vi "DFD Get Zero-Pole-Gain.vi"(7 "type (FLP)":enum16{"FLP", "FXP"}(ring), 8 "error in (no error)":errorcluster, 11 "filter in":T1={"mSRate_Fs"=1.0, "mSRate_Version"="2.0", "mSRate_Comments"="", "mSRate_OrgCoef"={"type"=enum."Undefined", "gain"=1.0, "coef a (k)"=[], "coef b (v)"=[]}, "mSRate_CurCoef"={"type"=enum."Undefined", "gain"=1.0, "coef a (k)"=[], "coef b (v)"=[]}, "mSRate_Quantized?"=FALSE, "mSRate_QCoef"={"type"=enum."Undefined", "gain"=1.0, "coef a (k)"=[], "coef b (v)"=[]}, "mSRate_QSettings"=[], "mSRate_Order"=0, "mSRate_Scaling"={"mSRate_ScaleByPowerOf2?"=FALSE, "mSRate_ScaleType"=enum."No Norm"}} {"mSRate_QSettings"."source" items=["Coef a/k"=0, "Coef b/v"=7, "Input"=1, "Output"=2, "Multiplicand"=3, "Product"=4, "Sum"=5, "Delay"=6, "Gain"=8]}) -> (0 "error out":errorcluster, 1 "poles":cdb[](array[numeric]) format="%.2f", 2 "zeroes":cdb[](array[numeric]) format="%.2f", 3 "filter out":T1={"mSRate_Fs"=1.0, "mSRate_Version"="2.0", "mSRate_Comments"="", "mSRate_OrgCoef"={"type"=enum."Undefined", "gain"=1.0, "coef a (k)"=[], "coef b (v)"=[]}, "mSRate_CurCoef"={"type"=enum."Undefined", "gain"=1.0, "coef a (k)"=[], "coef b (v)"=[]}, "mSRate_Quantized?"=FALSE, "mSRate_QCoef"={"type"=enum."Undefined", "gain"=1.0, "coef a (k)"=[], "coef b (v)"=[]}, "mSRate_QSettings"=[], "mSRate_Order"=0, "mSRate_Scaling"={"mSRate_ScaleByPowerOf2?"=FALSE, "mSRate_ScaleType"=enum."No Norm"}} {"mSRate_QSettings"."source" items=["Coef a/k"=0, "Coef b/v"=7, "Input"=1, "Output"=2, "Multiplicand"=3, "Product"=4, "Sum"=5, "Delay"=6, "Gain"=8]}, 5 "gain":dbl format="%.2f")   [LabVIEW 2017, in "NI_DigFilterLicensed.lvlib"]
doc: "Retrieves the zeroes, poles, and gain (ZPK) of a filter."
uses:
  <vilib>/addons/Digital Filter Design/NI_DigFilterLicensed.lvlib
  <vilib>/addons/Digital Filter Design/_Objects.llb/DFD Filter Obj.ctl
  <vilib>/addons/Digital Filter Design/_Objects.llb/DFD Filter Coef.ctl
  <vilib>/addons/Digital Filter Design/_Objects.llb/DFD Filter Structure Type Selector.ctl
  <vilib>/addons/Digital Filter Design/_Objects.llb/dfd_Internal Quantization Settings.ctl
  <vilib>/addons/Digital Filter Design/_Objects.llb/dfd_Internal Quantization Srcs.ctl
  <vilib>/addons/Digital Filter Design/_Objects.llb/DFD Coef Norm Type.ctl
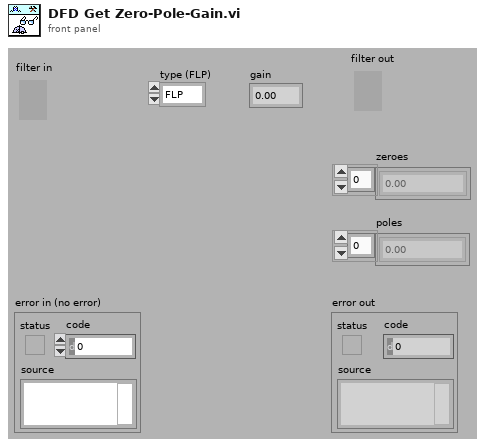
[diagram p1: front panel]
types:
  T1 = typedef "NI_DigFilterLicensed.lvlib/DFD Filter Obj.ctl" = cluster{"mSRate_Fs":dbl, "mSRate_Version":string, "mSRate_Comments":string, "mSRate_OrgCoef":T2, "mSRate_CurCoef":T2, "mSRate_Quantized?":bool, "mSRate_QCoef":T2, "mSRate_QSettings":T4[], "mSRate_Order":i32, "mSRate_Scaling":cluster{"mSRate_ScaleByPowerOf2?":bool, "mSRate_ScaleType":T6}}
  T2 = typedef "NI_DigFilterLicensed.lvlib/DFD Filter Coef.ctl" = cluster{"type":T3, "gain":dbl, "coef a (k)":dbl[], "coef b (v)":dbl[]}
  T3 = typedef "NI_DigFilterLicensed.lvlib/DFD Filter Structure Type Selector.ctl" = enum16{"Undefined", "FIR Direct Form", "FIR Direct Form Transposed", "FIR Symmetric", "FIR Antisymmetric", "IIR Direct Form I", "IIR Direct Form I Transposed", "IIR Direct Form II", "IIR Direct Form II Transposed", "IIR Cascaded Second Order Sections Form I", "IIR Cascaded Second Order Sections Form I Transposed", "IIR Cascaded Second Order Sections Form II", "IIR Cascaded Second Order Sections Form II Transposed", "Lattice Allpass (basic sections)", "Lattice Allpass (one multiplier sections)", "Lattice Allpass (normalized sections)", "Lattice AR (basic sections)", "Lattice AR (one multiplier sections)", "Lattice AR (normalized sections)", "Lattice MA (minimum phase)", "Lattice MA (maximum phase)", "Lattice ARMA (basic sections)", "Lattice ARMA (one multiplier sections)", "Lattice ARMA (normalized sections)"}
  T4 = typedef "NI_DigFilterLicensed.lvlib/dfd_Internal Quantization Settings.ctl" = cluster{"source":T5, "wl":i16, "iwl":i16, "overflow mode":enum16{"Saturation", "Wrap"}, "rounding mode":enum16{"Nearest", "Truncation"}, "signed?":bool}
  T5 = typedef "NI_DigFilterLicensed.lvlib/dfd_Internal Quantization Srcs.ctl" = u16
  T6 = typedef "NI_DigFilterLicensed.lvlib/DFD Coef Norm Type.ctl" = enum16{"No Norm", "Time Domain 1-Norm", "Time Domain 2-Norm", "Time Domain Inf-Norm"}
  T7 = typedef "NI_DigFilterLicensed.lvlib/DFD Filter Structure Id.ctl" = enum16{"Undefined", "FIR", "IIR Direct", "IIR SOS", "IIR Allpass", "IIR AR", "IIR ARMA"}
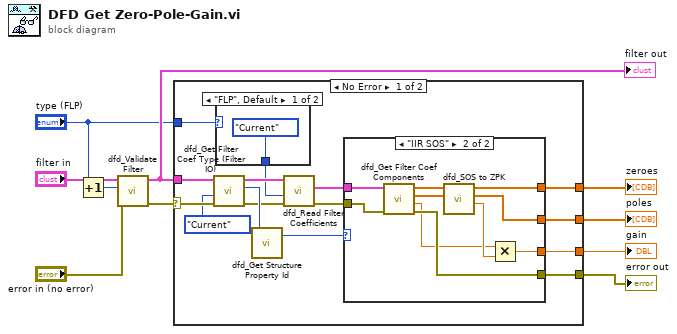
[diagram p0: block diagram]
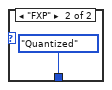
[diagram p2: hidden frame]
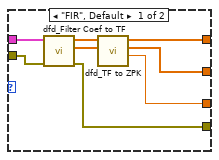
[diagram p3: hidden frame]
diagram:
  n1 = Increment(x="type (FLP)") -> (x+1=w2:enum16{"FLP", "FXP"})
  n2 = call <vilib>:"dfd_Validate Filter.vi"("error in (no error)"="error in (no error)", "check option"=w2, "filter in"="filter in") -> ("error out"=w3:errorcluster, "filter out"=w5:T1)  [unwired: 7 out]
  "filter out" <- w5
  n3 = case shown="No Error" w3 {
    selector: w3 -> [w19 w46]
    tunnel: w5 -> [w21 _]
    tunnel: [w25 _] -> w10
    tunnel: [w24 _] -> w9
    tunnel: [w23 _] -> w8
    tunnel: [w14 w46] -> w7
    tunnel: "type (FLP)" -> [w13 _]
    frame No Error {
      n4 = call <vilib>:"dfd_Get Filter Coef Type (Filter IO).vi"("error in (no error)"=w19, "coef source"=enum16{"Original", "Current", "Quantized"}."Current", "filter in"=w21) -> ("error out"=w17:errorcluster, "type"=w20:T3, "filter out"=w18:T1)  [unwired: 6 out]
      n5 = case shown="\"FLP\", Default" w13 {
        tunnel: [enum16{"Original", "Current", "Quantized"}."Current" ("coef source") enum16{"Original", "Current", "Quantized"}."Quantized" ("coef source")] -> w12
        frame "FLP", Default {
        }
        frame "FXP" {
        }
      }
      n6 = call <vilib>:"dfd_Get Structure Property Id.vi"("structure type"=w20) -> ("filter structure id"=w22:T7)  [unwired: 1 out]
      n7 = call <vilib>:"dfd_Read Filter Coefficients.vi"("error in (no error)"=w17, "coef source"=w12, "filter in"=w18) -> ("error out"=w15:errorcluster, "filter coef"=w16:T2)  [unwired: 7 out]
      n8 = case shown="\"IIR SOS\"" w22 {
        tunnel: [w35 w45] -> w25
        tunnel: [w33 w37] -> w24
        tunnel: [w34 w44] -> w23
        tunnel: w16 -> [w32 w42]
        tunnel: w15 -> [w31 w41]
        tunnel: [w30 w38] -> w14
        frame "FIR", Default {
          n9 = call <vilib>:"dfd_Filter Coef to TF.vi"("error out"=w31, "filter coef"=w32) -> ("error"=w30:errorcluster, "denominator"=w28:dbl[], "numerator"=w29:dbl[])  [unwired: 7 out]
          n10 = call <vilib>:"dfd_TF to ZPK.vi"("denominator"=w28, "numerator"=w29) -> ("gain"=w33:dbl, "poles"=w34:cdb[], "zeros"=w35:cdb[])  [unwired: 1 in, 6 out]
        }
        frame "IIR SOS" {
          n11 = call <vilib>:"dfd_Get Filter Coef Components.vi"("error in (no error)"=w41, "filter coef"=w42) -> ("error out"=w38:errorcluster, "gain"=w36:dbl, "coef a (k)"=w39:dbl[], "coef b (v)"=w40:dbl[])  [unwired: 6 out]
          n12 = call <vilib>:"dfd_SOS to ZPK.vi"("reverse coefficients"=w39, "forward coefficients"=w40) -> ("k"=w43:dbl, "poles"=w44:cdb[], "zeros"=w45:cdb[])  [unwired: 1 in, 6 out]
          n13 = Multiply(x=w36, y=w43) -> (x*y=w37:dbl)
        }
      }
    }
    frame Error {
    }
  }
  "zeroes" <- w10
  "poles" <- w8
  "gain" <- w9
  "error out" <- w7
